vi "ZCAN_Send&Receive.vi"(0 "can_index_handle":u32, 1 "ID":u32=18 format="0x%08x", 2 "Data":string="11 22 33 44 55 66 77 88", 5 "frame type":T1, 7 "agreement":T2, 9 "CANFD_SpeedUp":u32, 11 "error IO":errorcluster, 12 "milliseconds to wait":u32) -> (4 "Receive_Num":u32, 8 "CAN DATA":string, 15 "error out":errorcluster)   [LabVIEW 2020, in "zlgcan.lvlib"]
uses:
  zlgcan.lvlib
  data_type/Agreement.ctl
  data_type/frame type.ctl
  3eaebae9-40ef-4695-b156-7bc4e1103454.vi
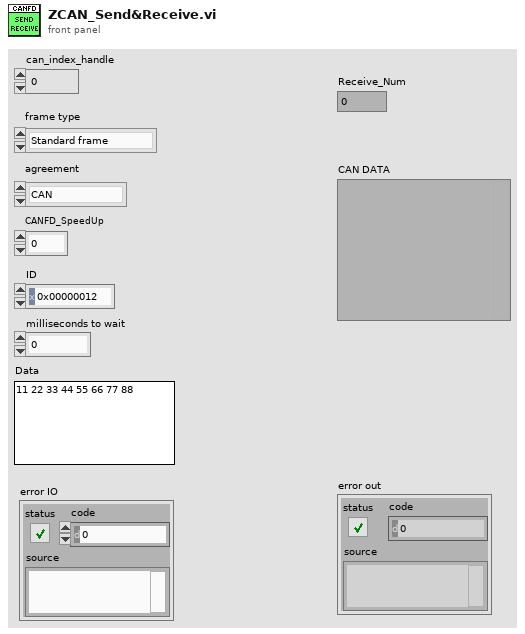
[diagram p1: front panel]
types:
  T1 = typedef "zlgcan.lvlib/frame type.ctl" = enum32{"Standard frame", "Extended frame"}
  T2 = typedef "zlgcan.lvlib/Agreement.ctl" = enum16{"CAN", "CANFD"}
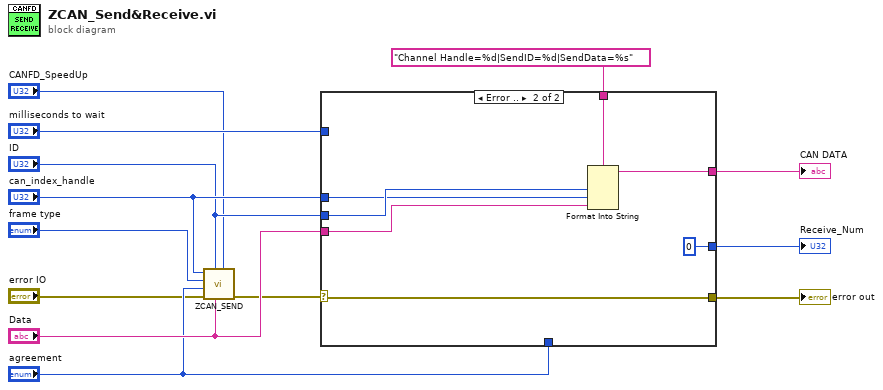
[diagram p0: block diagram]
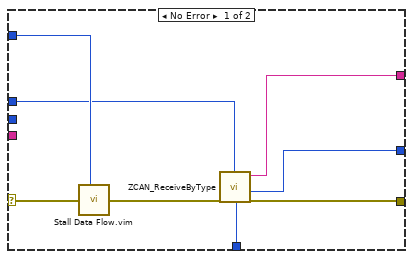
[diagram p2: hidden frame]
diagram:
  n1 = call "ZCAN_SEND.vi"("CANFD_SpeedUp"="CANFD_SpeedUp", "Data"="Data", "ID"="ID", "error IO"="error IO", "agreement"="agreement", "frame type"="frame type", "can_index_handle"="can_index_handle") -> ("error out"=w3:errorcluster)  [unwired: 4 in]
  n2 = case shown="Error .." w3 {
    selector: w3 -> [w14 w22]
    tunnel: "can_index_handle" -> [w16 w27]
    tunnel: [w20 w22] -> w8
    tunnel: [w17 w25] -> w7
    tunnel: "ID" -> [_ w28]
    tunnel: "Data" -> [_ w26]
    tunnel: "Channel Handle=%d|SendID=%d|SendData=%s" ("format string") -> [_ w24]
    tunnel: "milliseconds to wait" -> [w21 _]
    tunnel: [w18 u32 0 ("Receive_Num")] -> w5
    tunnel: "agreement" -> [w15 _]
    frame No Error {
      n3 = call "Stall Data Flow.vim"("value in"=w14, "milliseconds to wait"=w21) -> ("value out"=w19:errorcluster)  [unwired: 1 out]
      n4 = call "ZCAN_ReceiveByType.vi"("error in (no error)"=w19, "Agreement"=w15, "Can_CH_handle"=w16) -> ("error out"=w20:errorcluster, "Receive_Num"=w18:u32, "CAN DATA"=w17:string)  [unwired: 6 in]
    }
    frame Error {
      n5 = Format Into String(format string=w24, w28, w27, w26) -> (resulting string=w25:string)  [unwired: 2 in, 1 out]
    }
  }
  "error out" <- w8
  "CAN DATA" <- w7
  "Receive_Num" <- w5
